vi "WVFM_all.vi"(8 "dt":dbl, 10 "FPGA VI Reference":refnum<k20>) -> (1 "I array":waveform(sgl)[](array[waveform]), 2 "VR array":waveform(sgl)[](array[waveform]), 3 "VL array":waveform(sgl)[](array[waveform]))   [LabVIEW 2016]
uses:
  <vilib>/Utility/error.llb/Error Cluster From Error Code.vi
  <vilib>/rvi/errors/niLvFpgaAdjustHostInterfaceError.vi
  <vilib>/rvi/interface/nirviReadWriteControl/nirviReadWriteControl.xnode
  NiFpgaLv.dll
  <vilib>/rvi/interface/Simulation/niFpgaSimulationCallBeginRW.vi
panel:
  in  "waveform":waveform(sgl)
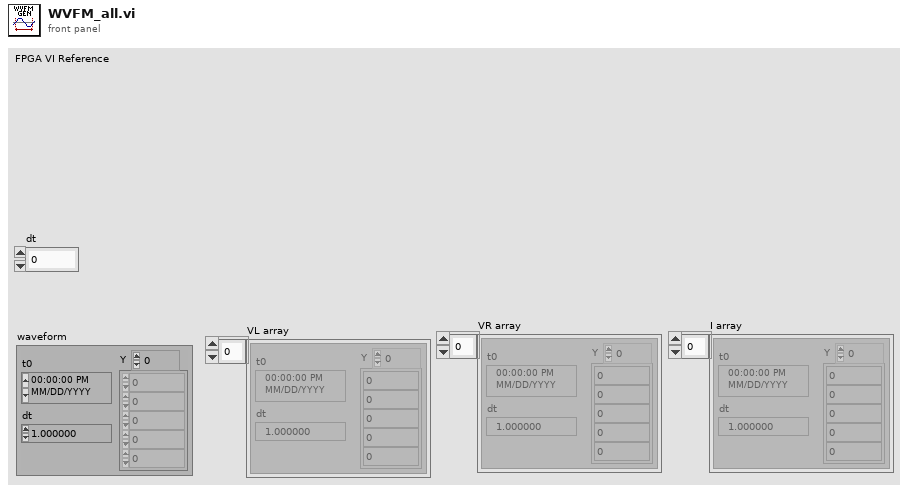
[diagram p1: front panel]
types:
  T1 = enum16{"Va L", "Vb L", "Vc L", "Ia", "Ib", "Ic", "Va R", "Vb R", "Vc R"}[]
  T2 = enum16{"Va L", "Vb L", "Vc L", "Ia", "Ib", "Ic", "Va R", "Vb R", "Vc R"}
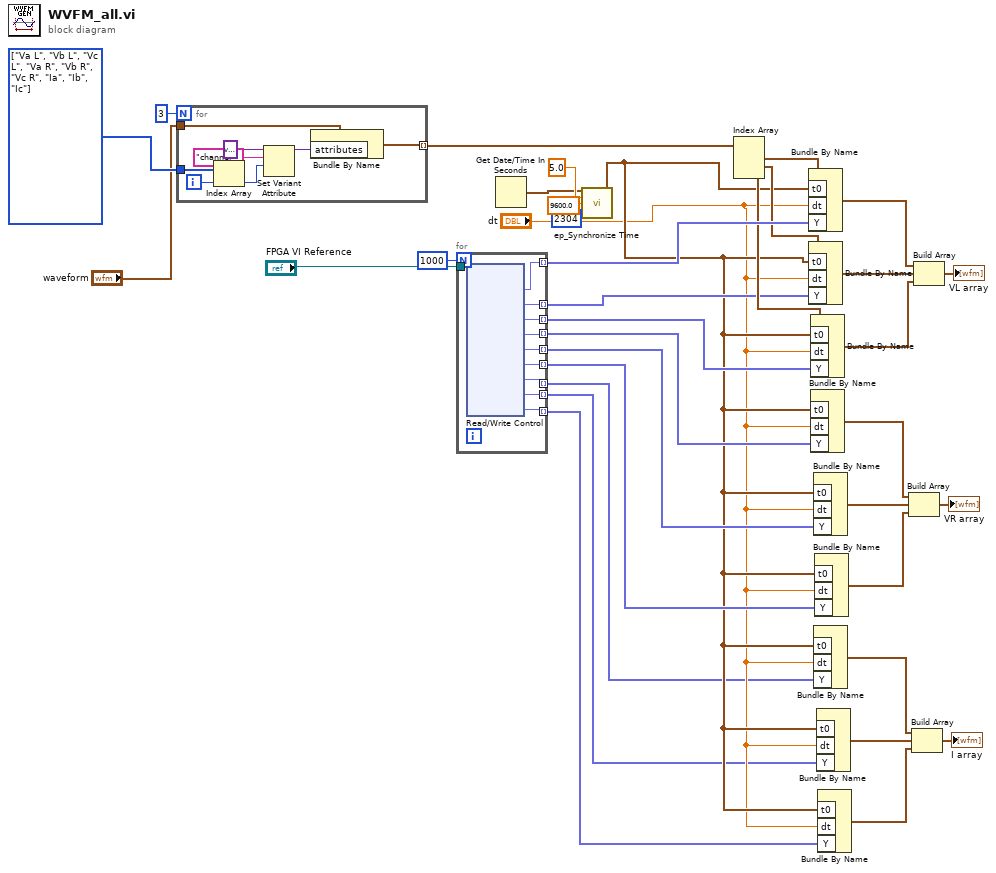
[diagram p0: block diagram]
diagram:
  w35 = T1 [enum."Va L", enum."Vb L", enum."Vc L", enum."Va R", enum."Vb R", enum."Vc R", enum."Ia", enum."Ib", enum."Ic"] items=["Va L", "Vb L", "Vc L", "Ia", "Ib", "Ic", "Va R", "Vb R", "Vc R"] ("Enum")
  n1 = for {
    N: 3 -> [_]
    tunnel: "waveform" -> [w39]
    tunnel: w35 -> [w42]
    tunnel: [w37] -> w34 mode=indexing
    i -> [w41]
    n2 = Index Array(array=w42, index=w41) -> (element=w40:T2)
    n3 = Set Variant Attribute(Variant=variant ("variant"), name="channel", value=w40) -> (Variant out=w38:variant)  [unwired: 1 in, 2 out]
    n4 = Bundle By Name(cluster=w39, "attributes"=w38) -> (w37:waveform(sgl))
  }
  n5 = for {
    N: 1000 -> [_]
    tunnel: "FPGA VI Reference" -> [w54]
    tunnel: [w53] -> w31 mode=indexing
    tunnel: [w52] -> w27 mode=indexing
    tunnel: [w51] -> w28 mode=indexing
    tunnel: [w50] -> w18 mode=indexing
    tunnel: [w49] -> w17 mode=indexing
    tunnel: [w48] -> w16 mode=indexing
    tunnel: [w47] -> w3 mode=indexing
    tunnel: [w46] -> w2 mode=indexing
    tunnel: [w45] -> w1 mode=indexing
    n6 = xnode "Read/Write Control"("FPGA VI Reference In"=w54) -> ("V7L AB"=w53:fxp<+/-,26,5>, "V7L BC"=w52:fxp<+/-,26,5>, "V7L CA"=w51:fxp<+/-,26,5>, "V7R AB"=w50:fxp<+/-,26,5>, "V7R BC"=w49:fxp<+/-,26,5>, "V7R CA"=w48:fxp<+/-,26,5>, "I7 A"=w47:fxp<+/-,26,5>, "I7 B"=w46:fxp<+/-,26,5>, "I7 C"=w45:fxp<+/-,26,5>)  [unwired: 1 in, 2 out]
  }
  n7 = Get Date/Time In Seconds() -> (seconds since 1Jan1904=w11:timestamp)
  n8 = call <vilib>:"ep_Synchronize Time.vi"("RT controler time in"=w11, "maximum time difference (sec)"=5.0, "sampling rate (Hz)"=9600.0, "basic calc. interval (samples)"=2304) -> ("RT controler time out"=w5:timestamp)  [unwired: 11 in]
  n9 = Index Array(array=w34) -> (element #1=w32:waveform(sgl), element #2=w30:waveform(sgl), element #3=w29:waveform(sgl))  [unwired: 3 in]
  n10 = Bundle By Name(cluster=w32, "t0"=w5, "dt"="dt", "Y"=w31) -> (w22:waveform(sgl))
  n11 = Bundle By Name(cluster=w30, "t0"=w5, "dt"="dt", "Y"=w27) -> (w21:waveform(sgl))
  n12 = Bundle By Name(cluster=w29, "t0"=w5, "dt"="dt", "Y"=w28) -> (w19:waveform(sgl))
  n13 = Bundle By Name("t0"=w5, "dt"="dt", "Y"=w18) -> (w15:waveform(sgl))  [unwired: 1 in]
  n14 = Bundle By Name("t0"=w5, "dt"="dt", "Y"=w17) -> (w14:waveform(sgl))  [unwired: 1 in]
  n15 = Bundle By Name("t0"=w5, "dt"="dt", "Y"=w3) -> (w6:waveform(sgl))  [unwired: 1 in]
  n16 = Bundle By Name("t0"=w5, "dt"="dt", "Y"=w16) -> (w13:waveform(sgl))  [unwired: 1 in]
  n17 = Bundle By Name("t0"=w5, "dt"="dt", "Y"=w2) -> (w7:waveform(sgl))  [unwired: 1 in]
  n18 = Bundle By Name("t0"=w5, "dt"="dt", "Y"=w1) -> (w8:waveform(sgl))  [unwired: 1 in]
  n19 = Build Array(w15, w14, w13) -> (→"VR array":waveform(sgl)[])
  n20 = Build Array(w6, w7, w8) -> (→"I array":waveform(sgl)[])
  n21 = Build Array(w22, w21, w19) -> (→"VL array":waveform(sgl)[])
